vi "Warning Judget.vi"(11 "Data In":string[](array[string])) -> (3 "Warning":bool)   [LabVIEW 2020]
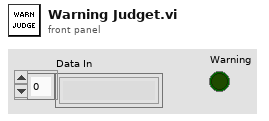
[diagram p1: front panel]
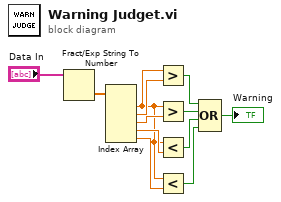
[diagram p0: block diagram]
diagram:
  n1 = Fract/Exp String To Number(string="Data In") -> (number=w12:dbl[])  [unwired: 3 in, 1 out]
  n2 = Index Array(array=w12) -> (element #1=w8:dbl, element #2=w11:dbl, element #3=w10:dbl, element #4=w9:dbl, element #5=w7:dbl)  [unwired: 5 in]
  n3 = Greater?(x=w8, y=w11) -> (0:w6:bool)
  n4 = Greater?(x=w8, y=w10) -> (0:w5:bool)
  n5 = Less?(x=w8, y=w9) -> (x < y?=w4:bool)
  n6 = Less?(x=w8, y=w7) -> (x < y?=w3:bool)
  n7 = Compound Arithmetic op=OR ("复合运算")(w6, w5, w4, w3) -> (→"Warning":bool)
